vi "Get Default Value.vi"(8 "error in":errorcluster, 9 "project refnum":refnum<vi>, 10 "measurement_signature":T2, 11 "gRPCid in":T1) -> (0 "error out":errorcluster, 3 "default value":variant)   [LabVIEW 2021, in "NI Measurement V2 Client Generator Runtime.lvlib"]
uses:
  NI Measurement V2 Client Generator Runtime.lvlib
  <vilib>/gRPC/Generated APIs/ni/measurementlink/measurement/v2/Measurement Service Client V2/RPC Messages/ni_measurementlink_measurement_v2_MeasurementSignature.ctl
  <vilib>/gRPC/Generated APIs/ni/measurementlink/measurement/v2/Measurement Service Client V2/RPC Messages/ni_measurementlink_measurement_v2_ConfigurationParameter.ctl
  <vilib>/gRPC/Generated APIs/ni/measurementlink/measurement/v2/Measurement Service Client V2/RPC Messages/google_protobuf_Field_Kind.ctl
  <vilib>/gRPC/Generated APIs/ni/measurementlink/measurement/v2/Measurement Service Client V2/RPC Messages/ni_measurementlink_measurement_v2_ConfigurationParameter_AnnotationsEntry.ctl
  <vilib>/gRPC/Generated APIs/ni/measurementlink/measurement/v2/Measurement Service Client V2/RPC Messages/google_protobuf_Any.ctl
  <vilib>/gRPC/Generated APIs/ni/measurementlink/measurement/v2/Measurement Service Client V2/RPC Messages/ni_measurementlink_measurement_v2_Output.ctl
  <vilib>/gRPC/Generated APIs/ni/measurementlink/measurement/v2/Measurement Service Client V2/RPC Messages/ni_measurementlink_measurement_v2_Output_AnnotationsEntry.ctl
  <vilib>/gRPC/LabVIEW gRPC Library/Shared/grpcId.ctl
  <vilib>/Utility/traverseref.llb/TRef TravTarget.ctl
  Client Generator Error Strings Global.vi
  <vilib>/gRPC/LabVIEW gRPC Library/grpc-lvsupport-release.lvlib
  <vilib>/Utility/traverseref.llb/VI Scripting - Traverse.lvlib
  <vilib>/gRPC/Generated APIs/ni/measurementlink/measurement/v2/Measurement Service Client V2/Measurement Service Client V2.lvlib
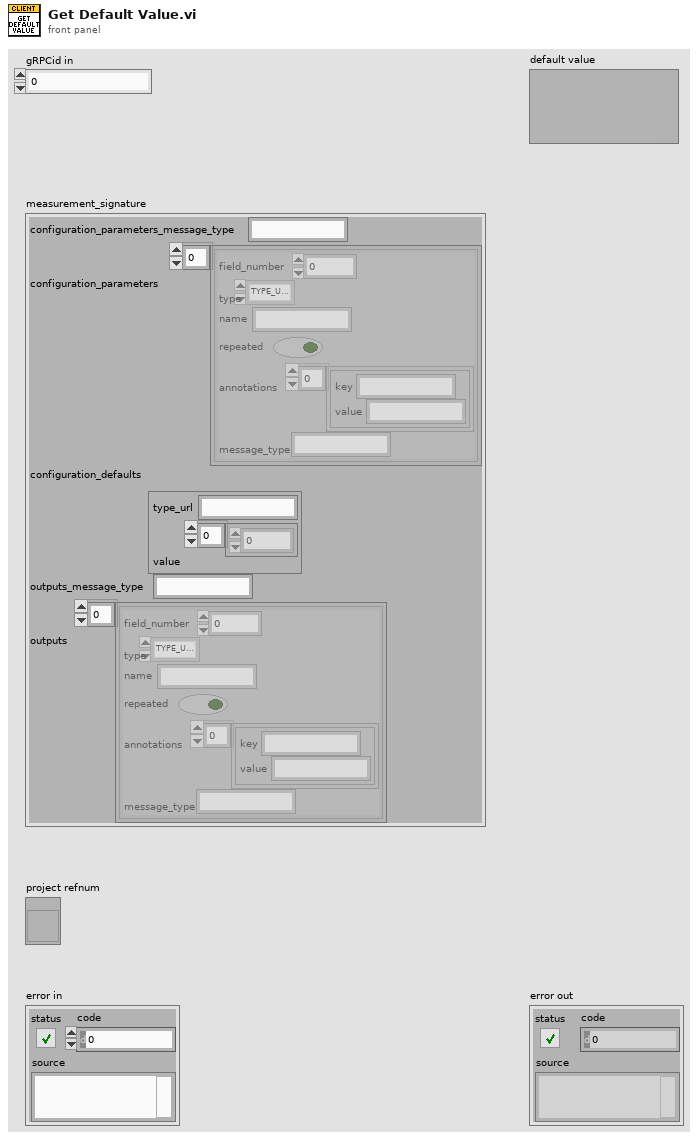
[diagram p1: front panel]
types:
  T1 = typedef "grpc-lvsupport-release.lvlib/grpcId.ctl" = u64
  T2 = typedef "Measurement Service Client V2.lvlib/ni_measurementlink_measurement_v2_MeasurementSignature.ctl" = cluster{"configuration_parameters_message_type":string, "configuration_parameters":T3[], "configuration_defaults":T6, "outputs_message_type":string, "outputs":T7[]}
  T3 = typedef "Measurement Service Client V2.lvlib/ni_measurementlink_measurement_v2_ConfigurationParameter.ctl" = cluster{"field_number":i32, "type":T4, "name":string, "repeated":bool, "annotations":T5[], "message_type":string}
  T4 = typedef "Measurement Service Client V2.lvlib/google_protobuf_Field_Kind.ctl" = enum32{"TYPE_UNKNOWN", "TYPE_DOUBLE", "TYPE_FLOAT", "TYPE_INT64", "TYPE_UINT64", "TYPE_INT32", "TYPE_FIXED64", "TYPE_FIXED32", "TYPE_BOOL", "TYPE_STRING", "TYPE_GROUP", "TYPE_MESSAGE", "TYPE_BYTES", "TYPE_UINT32", "TYPE_ENUM", "TYPE_SFIXED32", "TYPE_SFIXED64", "TYPE_SINT32", "TYPE_SINT64"}
  T5 = typedef "Measurement Service Client V2.lvlib/ni_measurementlink_measurement_v2_ConfigurationParameter_AnnotationsEntry.ctl" = cluster{"key":string, "value":string}
  T6 = typedef "Measurement Service Client V2.lvlib/google_protobuf_Any.ctl" = cluster{"type_url":string, "value":u8[]}
  T7 = typedef "Measurement Service Client V2.lvlib/ni_measurementlink_measurement_v2_Output.ctl" = cluster{"field_number":i32, "type":T4, "name":string, "repeated":bool, "annotations":T8[], "message_type":string}
  T8 = typedef "Measurement Service Client V2.lvlib/ni_measurementlink_measurement_v2_Output_AnnotationsEntry.ctl" = cluster{"key":string, "value":string}
  T9 = typedef "TRef TravTarget.ctl" = enum16{"FP", "BD", "Other"}
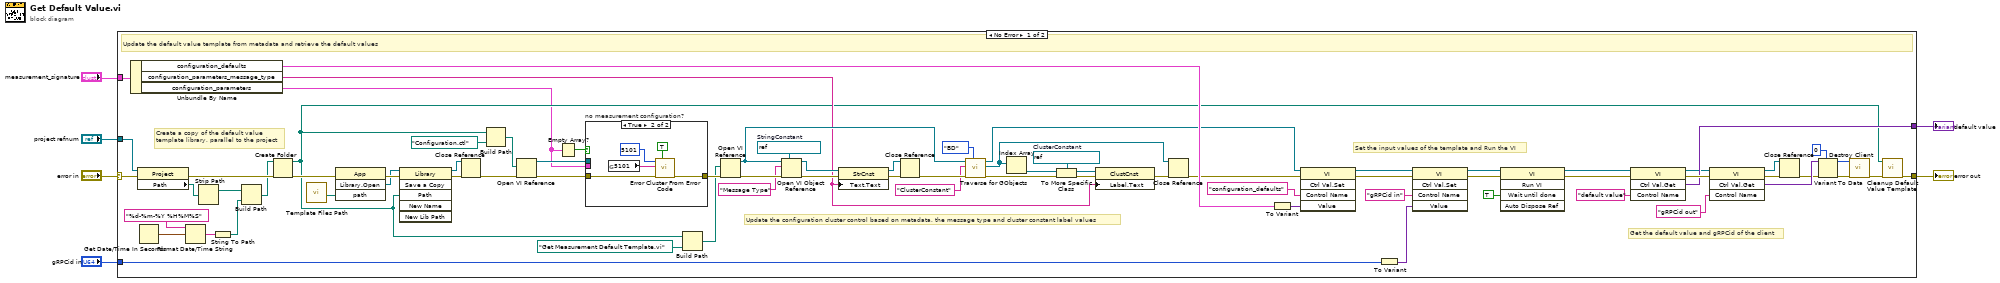
[diagram p0: block diagram]
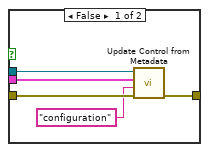
[diagram p2: hidden frame]
diagram:
  n1 = case shown="No Error" "error in" {
    selector: "error in" -> [w82 w93]
    tunnel: [w19 w93] -> w5
    tunnel: "measurement_signature" -> [w7 _]
    tunnel: "gRPCid in" -> [w66 _]
    tunnel: [w57 _] -> w2
    tunnel: "project refnum" -> [w39 _]
    frame No Error {
      w44 = refnum<vi> refnum  # ClusterConstant
      w77 = refnum<vi> refnum  # StringConstant
      # "Get the default value and gRPCid of the client"
      # "Set the input values of the template and Run the VI"
      # "Update the configuration cluster control based on metadata, the message type and cluster constant label values"
      # "Create a copy of the default value\ntemplate library, parallel to the project"
      # "Update the default value template from metadata and retrieve the default values"
      n2 = Unbundle By Name(w7) -> ("configuration_defaults"=w70:T6, "configuration_parameters_message_type"=w41:string, "configuration_parameters"=w8:T3[])
      n3 = property class="Project"(reference=w39, error in=w82) -> (error out=w35:errorcluster, "Path"=w38:path)  [unwired: 1 out]
      n4 = Get Date/Time In Seconds() -> (seconds since 1Jan1904=w37:timestamp)
      n5 = Format Date/Time String(time format string (%c)="%d-%m-%Y %H%M%S", seconds (now)=w37) -> (date/time string=w11:string)  [unwired: 1 in]
      n6 = Strip Path(path=w38) -> (stripped path=w36:path)  [unwired: 1 out]
      n7 = String To Path(string=w11) -> (path=w10:path)
      n8 = Build Path(base path=w36, name or relative path=w10) -> (appended path=w33:path)
      n9 = Create Folder(path (use dialog)=w33, error in=w35) -> (created path=w17:path, error out=w34:errorcluster)  [unwired: 1 in, 1 out]
      n10 = call "Template Files Path.vi"() -> ("default template path"=w20:path)  [unwired: 9 in, 2 out]
      n11 = invoke class="App" method="Library.Open"(error in=w34, "path"=w20) -> (error out=w26:errorcluster, "Open Library"=w24:refnum<vi>)  [unwired: 2 in, 2 out]
      n12 = invoke class="Library" method="Save a Copy"(reference=w24, error in=w26, "Path"=w17) -> (reference out=w21:refnum<vi>, error out=w25:errorcluster)  [unwired: 3 in, 4 out]
      n13 = Close Reference(reference=w21, error in (no error)=w25) -> (error out=w22:errorcluster)
      n14 = Build Path(base path=w17, name or relative path=path "Configuration.ctl") -> (appended path=w31:path)
      n15 = Open VI Reference(vi path=w31, error in (no error)=w22) -> (vi reference=w30:refnum<vi>, error out=w32:errorcluster)  [unwired: 4 in]
      n16 = Empty Array?(array=w8) -> (empty?=w9:bool)
      n17 = case "no measurement configuration?" shown="True" w9 {
        tunnel: [w87 w91] -> w81
        tunnel: w32 -> [w86 w92]
        tunnel: w30 -> [w85 _]
        tunnel: w8 -> [w83 _]
        frame False {
          n18 = call "Update Control from Metadata.vi"("error in"=w86, "control name"="configuration", "parameter data"=w83, "vi refnum"=w85) -> ("error out"=w87:errorcluster)  [unwired: 7 in]
        }
        frame True {
          n19 = global read "Client Generator Error Strings Global.vi" "5101"() -> (w89:string)
          n20 = call <vilib>:"Error Cluster From Error Code.vi"("show call chain? (False)"=TRUE, "error in (no error)"=w92, "error message (\"\")"=w89, "error code (0)"=5101) -> ("error out"=w91:errorcluster)  [unwired: 5 in]
        }
      }
      n21 = Build Path(base path=w17, name or relative path=path "Get Measurement Default Template.vi") -> (appended path=w28:path)
      n22 = Open VI Reference(vi path=w28, error in (no error)=w81) -> (vi reference=w48:refnum<vi>, error out=w80:errorcluster)  [unwired: 4 in]
      n23 = Open VI Object Reference(7:w77, 8:w80, 10:"Message Type" ("name/order"), 11:w48) -> (0:w78:errorcluster, 3:w75:refnum<vi>)
      n24 = property class="StrCnst"(reference=w75, error in=w78, "Text.Text"=w41) -> (reference out=w74:refnum<vi>, error out=w76:errorcluster)
      n25 = Close Reference(reference=w74, error in (no error)=w76) -> (error out=w73:errorcluster)
      n26 = call <vilib>:"Traverse for GObjects.vi"("Traverse Target"=TRef_TravTarget."BD", "error in (no error)"=w73, "Class Name"="ClusterConstant", "VI Refnum"=w48) -> ("error out"=w45:errorcluster, "References"=w18:refnum<vi>[], "dup VI Refnum"=w51:refnum<vi>)  [unwired: 4 in, 1 out]
      n27 = Index Array(array=w18) -> (element=w43:refnum<vi>)  [unwired: 1 in]
      n28 = To More Specific Class(target class=w44, reference=w43, error in=w45) -> (specific class reference=w42:refnum<vi>, error out=w46:errorcluster)
      n29 = property class="ClustCnst"(reference=w42, error in=w46, "Label.Text"=w41) -> (error out=w47:errorcluster)  [unwired: 1 out]
      n30 = Close Reference(reference=w18, error in (no error)=w47) -> (error out=w40:errorcluster)
      n31 = To Variant(anything=w70) -> (Variant=w69:variant)
      n32 = invoke class="VI" method="Ctrl Val.Set"(reference=w51, error in=w40, "Control Name"="configuration_defaults", "Value"=w69) -> (reference out=w67:refnum<vi>, error out=w72:errorcluster)  [unwired: 1 in, 3 out]
      n33 = To Variant(anything=w66) -> (Variant=w65:variant)
      n34 = invoke class="VI" method="Ctrl Val.Set"(reference=w67, error in=w72, "Control Name"="gRPCid in", "Value"=w65) -> (reference out=w62:refnum<vi>, error out=w68:errorcluster)  [unwired: 1 in, 3 out]
      n35 = invoke class="VI" method="Run VI"(reference=w62, error in=w68, "Wait until done"=TRUE ("Wait Until Done")) -> (reference out=w59:refnum<vi>, error out=w63:errorcluster)  [unwired: 2 in, 3 out]
      n36 = invoke class="VI" method="Ctrl Val.Get"(reference=w59, error in=w63, "Control Name"="default value") -> (reference out=w55:refnum<vi>, error out=w60:errorcluster, "Get Control Value Variant"=w57:variant)  [unwired: 1 in, 1 out]
      n37 = invoke class="VI" method="Ctrl Val.Get"(reference=w55, error in=w60, "Control Name"="gRPCid out") -> (reference out=w13:refnum<vi>, error out=w56:errorcluster, "Get Control Value Variant"=w53:variant)  [unwired: 1 in, 1 out]
      n38 = Close Reference(reference=w13, error in (no error)=w56) -> (error out=w14:errorcluster)
      n39 = Variant To Data(error in=w14, type=T1 0 ("gRPCid in"), Variant=w53) -> (data=w12:T1, error out=w15:errorcluster)
      n40 = call <vilib>:"Destroy Client.vi"("error in"=w15, "gRPC ID"=w12) -> ("error out"=w16:errorcluster)  [unwired: 9 in]
      n41 = call "Cleanup Default Value Template.vi"("error in"=w16, "temporary template path"=w17) -> ("error out"=w19:errorcluster)  [unwired: 9 in]
    }
    frame Error {
      # "Pass"
    }
  }
  "error out" <- w5
  "default value" <- w2
